vi "PM5000_VIFP_Main.vi"(8 "error in":errorcluster, 11 "Network Path In":string="172.22.26.202") -> (0 "error out":errorcluster, 2 "VIFP_Main out":T1, 3 "Network Path Out":string="192.168.169.1")   [LabVIEW 2018]
doc: "Lee la tabla de memoria RealTime_VIF_Power del equipo PowerMonitor 5000, ademas filtra y ordena las variables de interez de la tabla de memoria.\n\nLee las siguientes variables de la tabla RealTime_VIF_Power:\n\n* Avg_VL_VL_Volts\n* Avg_Amps\n* Avg_Frequency_Hz\n* Total_kW"
uses:
  <vilib>/ethernetip/ethernetip.llb/EthernetIP SLC500 Read Float.vi
  <vilib>/ethernetip/ethernetip.lvlib
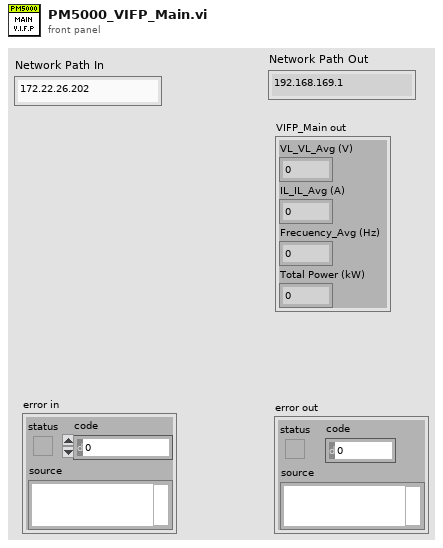
[diagram p1: front panel]
types:
  T1 = cluster{"VL_VL_Avg (V)":sgl, "IL_IL_Avg (A)":sgl, "Frecuency_Avg (Hz)":sgl, "Total Power (kW)":sgl}
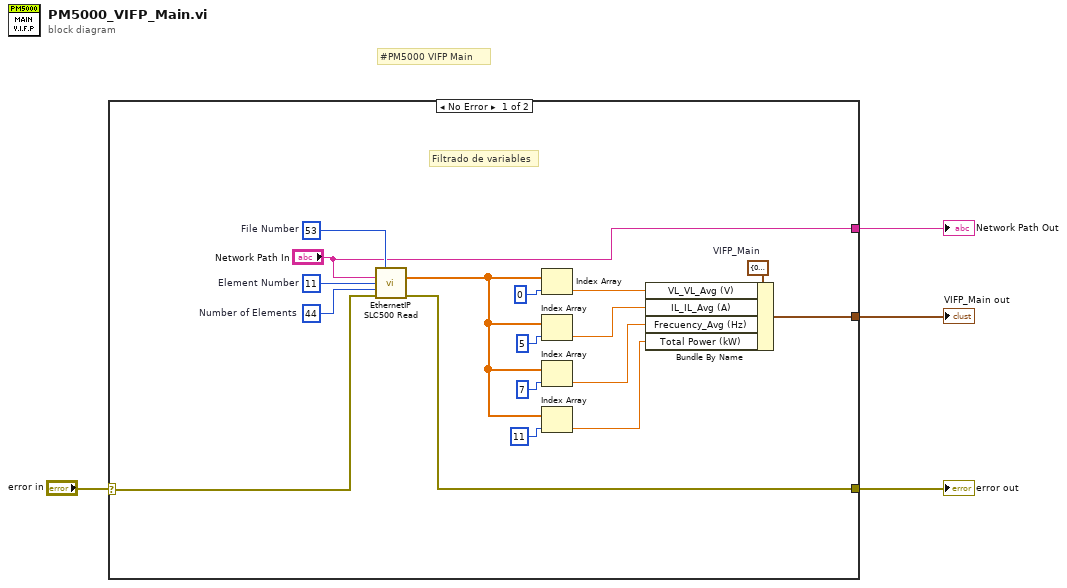
[diagram p0: block diagram]
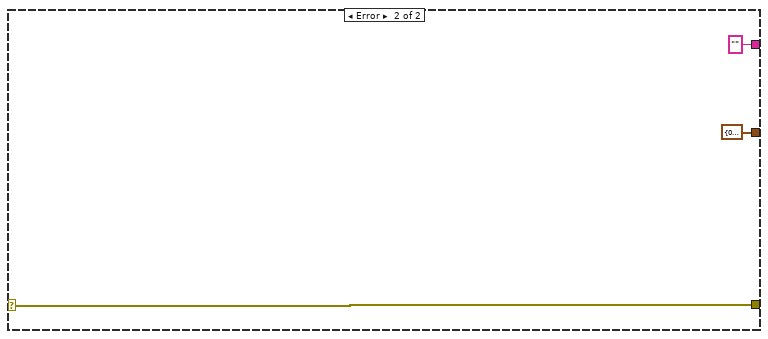
[diagram p2: hidden frame]
diagram:
  # "#PM5000 VIFP Main"
  n1 = case shown="No Error" "error in" {
    selector: "error in" -> [w12 w24]
    tunnel: [w18 w24] -> w4
    tunnel: ["Network Path In" "" ("Network Path In")] -> w2
    tunnel: [w5 T1 {"VL_VL_Avg (V)"=0.0, "IL_IL_Avg (A)"=0.0, "Frecuency_Avg (Hz)"=0.0, "Total Power (kW)"=0.0} ("VIFP_Main")] -> w1
    frame No Error {
      w11 = T1 {"VL_VL_Avg (V)"=0.0, "IL_IL_Avg (A)"=0.0, "Frecuency_Avg (Hz)"=0.0, "Total Power (kW)"=0.0}  # VIFP_Main
      w19 = u32 44  # Number of Elements
      w21 = u16 53  # File Number
      w20 = u16 11  # Element Number
      # "Filtrado de variables"
      n2 = call-poly <vilib>:"EthernetIP SLC500 Read.vi"("File Number"=w21, "Network Path"="Network Path In", "Element Number"=w20, "Number of Elements"=w19, "error in"=w12) -> ("Data"=w17:sgl[], "error out"=w18:errorcluster)  [unwired: 8 in, 1 out]
      n3 = Index Array(array=w17, index=0) -> (element=w10:sgl)
      n4 = Index Array(array=w17, index=5) -> (element=w9:sgl)
      n5 = Index Array(array=w17, index=7) -> (element=w8:sgl)
      n6 = Index Array(array=w17, index=11) -> (element=w7:sgl)
      n7 = Bundle By Name(cluster=w11, "VL_VL_Avg (V)"=w10, "IL_IL_Avg (A)"=w9, "Frecuency_Avg (Hz)"=w8, "Total Power (kW)"=w7) -> (w5:T1)
    }
    frame Error {
    }
  }
  "error out" <- w4
  "Network Path Out" <- w2
  "VIFP_Main out" <- w1
